vi "OldDemo.vi"() -> ()   [LabVIEW 2020]
uses:
  ReadOnshapeAngle.vi
  WriteOnshapeAngle.vi
panel:
  out "Angle1 Out":dbl
  out "Angle2 Out":dbl
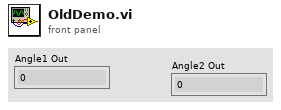
[diagram p1: front panel]
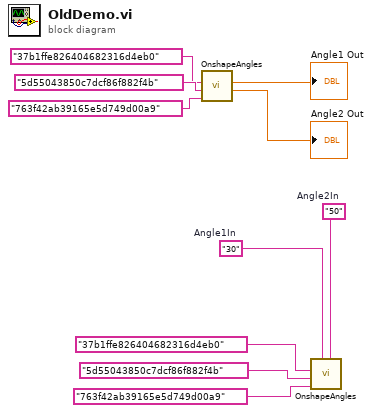
[diagram p0: block diagram]
diagram:
  w9 = "50"  # Angle2In
  w8 = "30"  # Angle1In
  n1 = call-poly "OnshapeAngles.vi"("eid"="763f42ab39165e5d749d00a9", "wid"="5d55043850c7dcf86f882f4b", "did"="37b1ffe826404682316d4eb0") -> ("Angle2Out"=→"Angle2 Out":dbl, "Angle1Out"=→"Angle1 Out":dbl)  [unwired: 6 in, 1 out]
  n2 = call-poly "OnshapeAngles.vi"("Angle2In"=w9, "Angle1In"=w8, "eid"="763f42ab39165e5d749d00a9", "wid"="5d55043850c7dcf86f882f4b", "did"="37b1ffe826404682316d4eb0") -> ()  [unwired: 6 in, 1 out]
